vi "Add Wheels to Steering Frame.vi"   [LabVIEW 2017, in "NI_Robotics_Steering Frame.lvclass"]
doc: "Adds the wheel or wheels you specify to <B>steering frame in</B>. You must manually select the polymorphic instance to use."
uses:
  <vilib>/robotics/Steering/Steering Frame/NI_Robotics_Steering Frame.lvclass
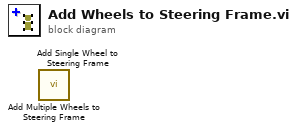
[diagram p0: block diagram]
diagram:
  n1 = call <vilib>:"Add Multiple Wheels to Steering Frame.vi"() -> ()  [unwired: 10 in, 2 out]
  n2 = call <vilib>:"Add Single Wheel to Steering Frame.vi"() -> ()  [unwired: 10 in, 2 out]
